vi "_Import Permanent Variable.vi"(7 "in":T3, 8 "error in (no error)":errorcluster, 9 "Array":path[](array[path]), 10 "section postfix":string, 11 "Path":path) -> (0 "error out":errorcluster, 5 "out":T3)   [LabVIEW 2017, in "INI-Static-Variable-Support.lvlib" / "CSM-Static-Variable-Manager.lvclass"]
uses:
  CSM-Static-Variable-Manager.lvclass
  LabVIEW-Config/Config.ctl
  LabVIEW-Config/LineToken.ctl
  LabVIEW-Config/LabVIEW-Config.lvlib
  <userlib>/_NEVSTOP/Communicable State Machine(CSM)/addons/API-String-Arugments-Support/API String Arguments Support.lvlib
  <userlib>/_NEVSTOP/Communicable State Machine(CSM)/_Shared/CSM Shared.lvlib
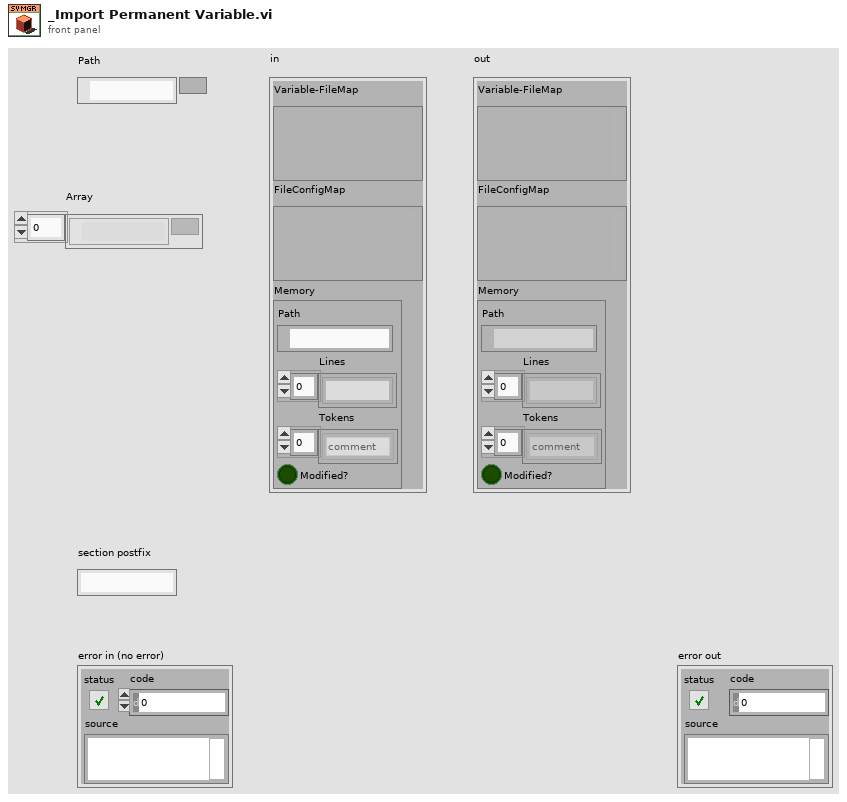
[diagram p1: front panel]
types:
  T1 = typedef "LabVIEW-Config.lvlib/Config.ctl" = cluster{"Path":path, "Lines":string[], "Tokens":T2[], "Modified?":bool}
  T2 = typedef "LabVIEW-Config.lvlib/LineToken.ctl" = enum8{"comment", "section", "key", "more"}
  T3 = cluster{"Variable-FileMap":variant, "FileConfigMap":variant, "Memory":T1}
  T4 = enum16{"Absolute path", "Relative path", "Not-a-path"}
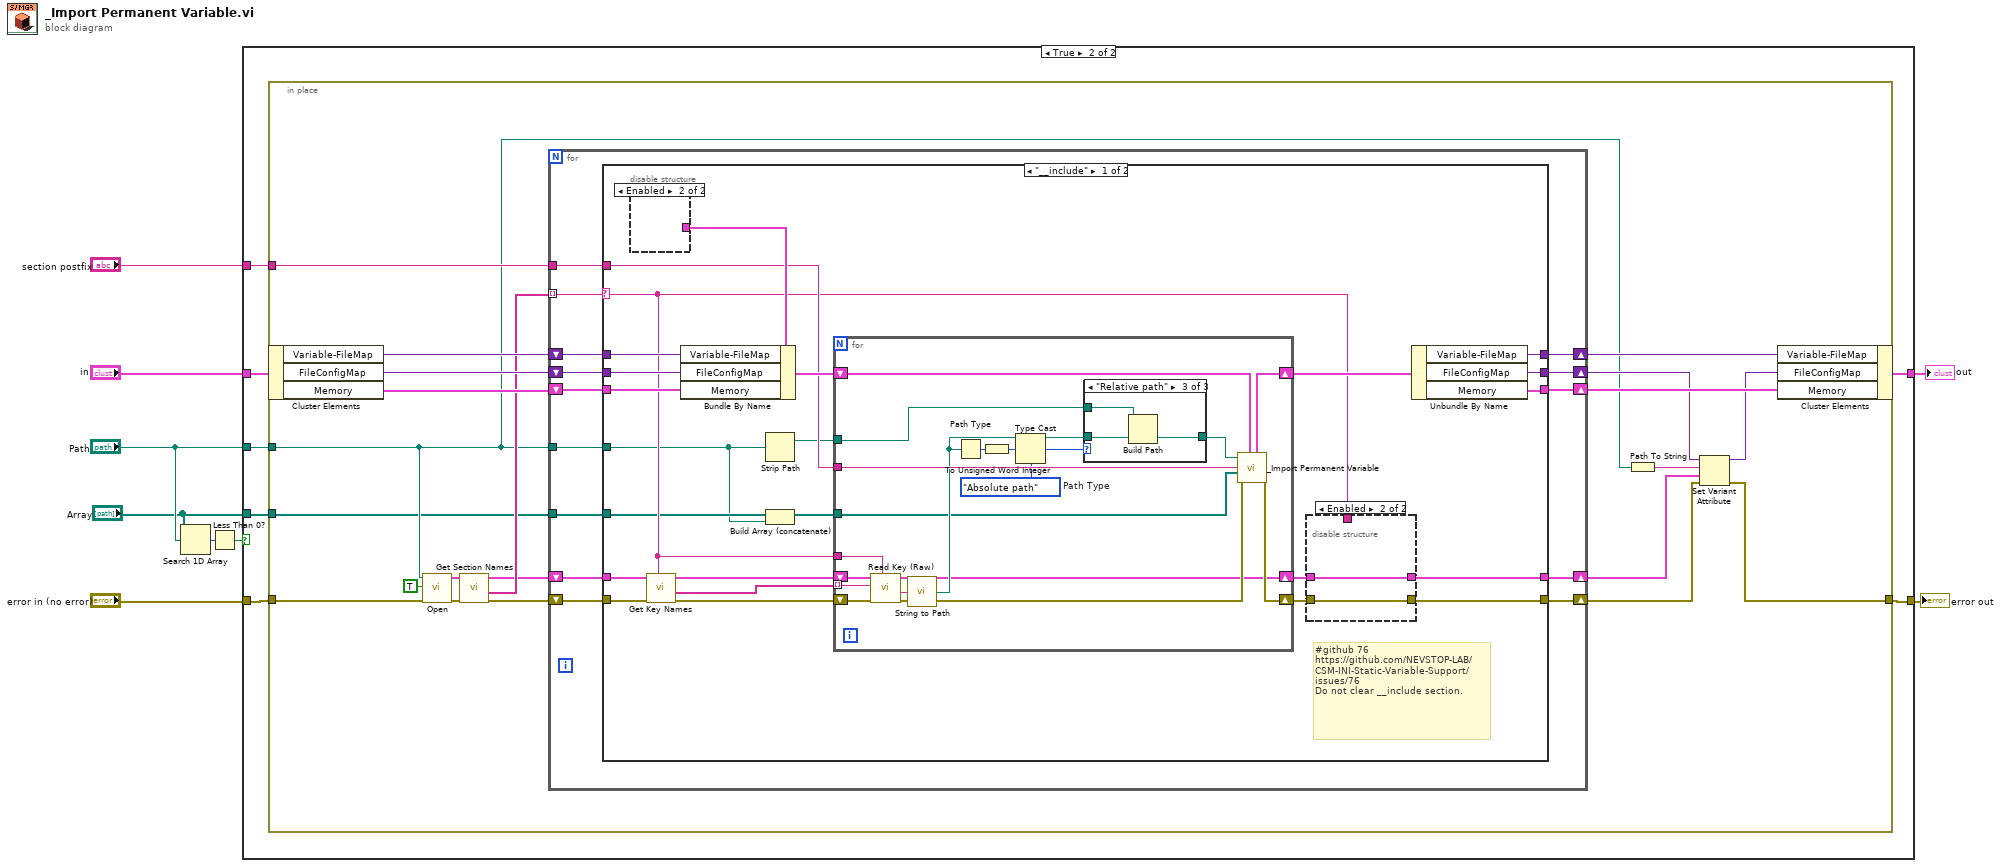
[diagram p0: block diagram]
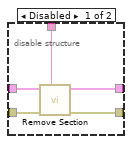
[diagram p3: hidden frame]
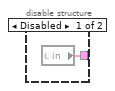
[diagram p6: hidden frame]
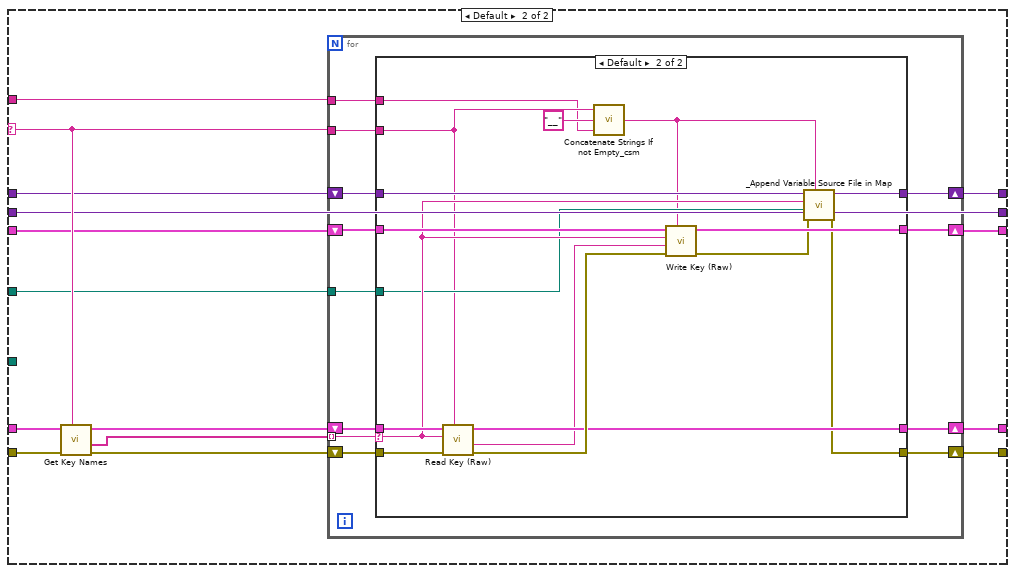
[diagram p7: hidden frame]
diagram:
  n1 = Search 1D Array(1D array="Array", element="Path") -> (index of element=w3:i32)  [unwired: 1 in]
  n2 = Less Than 0?(x=w3) -> (x < 0?=w2:bool)
  n3 = case shown="True" w2 {
    tunnel: "Path" -> [_ w18]
    tunnel: [w10 w17] -> w8
    tunnel: "section postfix" -> [_ w16]
    tunnel: "in" -> [w11 w15]
    tunnel: [w11 w14] -> w5
    tunnel: "error in (no error)" -> [w10 w13]
    tunnel: "Array" -> [_ w12]
    frame False {
    }
    frame True {
      n4 = in-place {
        in-place-border: w18 -> [w20]
        in-place-border: [w28] -> w17
        in-place-border: w16 -> [w39]
        in-place-border: w13 -> [w25]
        in-place-border: w12 -> [w19]
        n5 = in-place-cluster #1(w15) -> ("Variable-FileMap"=w38:variant, "FileConfigMap"=w34:variant, "Memory"=w37:T1)
        n6 = call "Open.vi"("error in (no error)"=w25, "Create if not exists? (T)"=TRUE, "Path"=w20) -> ("error out"=w27:errorcluster, "Config"=w26:T1)  [unwired: 5 in, 2 out]
        n7 = call "Get Section Names.vi"("error in (no error)"=w27, "Config in"=w26) -> ("error out"=w23:errorcluster, "Section Names"=w22:string[], "Config out"=w21:T1)  [unwired: 7 in]
        n8 = for {
          tunnel: w22 -> [w51] mode=indexing
          shift-right: [w49] -> w35
          shift-left: w37 -> [w50]
          shift-right: [w48] -> w29
          shift-left: w23 -> [w52]
          shift-right: [w47] -> w30
          shift-left: w21 -> [w53]
          shift-right: [w46] -> w36
          shift-left: w38 -> [w45]
          tunnel: w20 -> [w44]
          tunnel: w39 -> [w43]
          shift-right: [w42] -> w32
          shift-left: w34 -> [w41]
          tunnel: w19 -> [w40]
          n9 = case shown="\"__include\"" w51 {
            selector: w51 -> [w57 w122]
            tunnel: w53 -> [w65 w124]
            tunnel: w52 -> [w66 w123]
            tunnel: w50 -> [w73 w118]
            tunnel: [w70 w117] -> w49
            tunnel: [w60 w116] -> w48
            tunnel: [w58 w115] -> w47
            tunnel: [w68 w114] -> w46
            tunnel: w45 -> [w75 w113]
            tunnel: w44 -> [w54 w112]
            tunnel: w43 -> [w67 w111]
            tunnel: [w69 w110] -> w42
            tunnel: w41 -> [w74 w110]
            tunnel: w40 -> [w56 _]
            frame "__include" {
              # "#github 76\nhttps://github.com/NEVSTOP-LAB/CSM-INI-Static-Variable-Support/issues/76\nDo not clear __include section."
              n10 = disable-structure shown="Enabled" {
                disable-tunnel: [w109 _] -> w76
                frame Disabled {
                  n11 = local read "in"() -> (w109:T3)
                }
                frame Enabled {
                }
              }
              n12 = call "Get Key Names.vi"("Section Name"=w57, "error in (no error)"=w66, "Config in"=w65) -> ("error out"=w63:errorcluster, "Key Names"=w61:string[], "Config out"=w64:T1)  [unwired: 5 in, 1 out]
              n13 = Bundle By Name(cluster=w76, "Variable-FileMap"=w75, "FileConfigMap"=w74, "Memory"=w73) -> (w72:T3)
              n14 = Strip Path(path=w54) -> (stripped path=w62:path)  [unwired: 1 out]
              n15 = Build Array (concatenate)(w56, w54) -> (w55:path[])
              n16 = for {
                tunnel: w67 -> [w100]
                shift-right: [w103] -> w77
                shift-left: w63 -> [w96]
                shift-right: [w101] -> w71
                shift-left: w72 -> [w102]
                shift-right: [w91] -> w59
                shift-left: w64 -> [w97]
                tunnel: w62 -> [w98]
                tunnel: w61 -> [w95] mode=indexing
                tunnel: w57 -> [w90]
                tunnel: w55 -> [w89]
                w87 = T4."Absolute path"  # Path Type
                n17 = call "Read Key (Raw).vi"("Section Name"=w90, "error in (no error)"=w96, "Key Name"=w95, "Config in"=w97) -> ("error out"=w94:errorcluster, "Content"=w93:string, "Config out"=w91:T1)  [unwired: 4 in, 1 out]
                n18 = call <userlib>:"String to Path.vi"("String"=w93) -> ("Path"=w92:path)
                n19 = Path Type(1:w92) -> (0:w88:i16)
                n20 = To Unsigned Word Integer(number=w88) -> (unsigned 16bit integer=w86:u16)
                n21 = Type Cast(type=w87, x=w86) -> (*(type *) &x=w85:T4)
                n22 = case shown="\"Relative path\"" w85 {
                  tunnel: w92 -> [w104 w105 w107]
                  tunnel: [w104 w105 w106] -> w99
                  tunnel: w98 -> [_ _ w108]
                  frame "Absolute path" {
                  }
                  frame "Not-a-path" {
                  }
                  frame "Relative path" {
                    n23 = Build Path(base path=w108, name or relative path=w107) -> (appended path=w106:path)
                  }
                }
                n24 = call "_Import Permanent Variable.vi"("in"=w102, "error in (no error)"=w94, "Array"=w89, "section postfix"=w100, "Path"=w99) -> ("error out"=w103:errorcluster, "out"=w101:T3)  [unwired: 5 in]
              }
              n25 = disable-structure shown="Enabled" {
                disable-tunnel: w77 -> [w82 w83]
                disable-tunnel: [w81 w83] -> w60
                disable-tunnel: w59 -> [w80 w84]
                disable-tunnel: [w79 w84] -> w58
                disable-tunnel: w57 -> [w78 _]
                frame Disabled {
                  n26 = call "Remove Section.vi"("Section Name"=w78, "error in (no error)"=w82, "Config in"=w80) -> ("error out"=w81:errorcluster, "Config out"=w79:T1)  [unwired: 6 in, 1 out]
                }
                frame Enabled {
                }
              }
              n27 = Unbundle By Name(w71) -> ("Variable-FileMap"=w68:variant, "FileConfigMap"=w69:variant, "Memory"=w70:T1)
            }
            frame Default {
              n28 = call "Get Key Names.vi"("Section Name"=w122, "error in (no error)"=w123, "Config in"=w124) -> ("error out"=w119:errorcluster, "Key Names"=w120:string[], "Config out"=w121:T1)  [unwired: 5 in, 1 out]
              n29 = for {
                tunnel: w122 -> [w126]
                tunnel: w120 -> [w128] mode=indexing
                shift-right: [w130] -> w116
                shift-left: w119 -> [w135]
                shift-right: [w134] -> w117
                shift-left: w118 -> [w133]
                shift-right: [w132] -> w115
                shift-left: w121 -> [w136]
                shift-right: [w131] -> w114
                shift-left: w113 -> [w129]
                tunnel: w112 -> [w127]
                tunnel: w111 -> [w125]
                n30 = case shown="Default" w128 {
                  selector: w128 -> [_ w146]
                  tunnel: w136 -> [w138 w157]
                  tunnel: w135 -> [w137 w156]
                  tunnel: [w139 w155] -> w134
                  tunnel: w133 -> [w139 w154]
                  tunnel: [w138 w152] -> w132
                  tunnel: [w140 w151] -> w131
                  tunnel: [w137 w149] -> w130
                  tunnel: w129 -> [w140 w148]
                  tunnel: w127 -> [_ w145]
                  tunnel: w126 -> [_ w142]
                  tunnel: w125 -> [_ w141]
                  frame "Core.Current VI Reference" {
                  }
                  frame Default {
                    n31 = call "Read Key (Raw).vi"("Section Name"=w142, "error in (no error)"=w156, "Key Name"=w146, "Config in"=w157) -> ("error out"=w153:errorcluster, "Content"=w147:string, "Config out"=w152:T1)  [unwired: 4 in, 1 out]
                    n32 = call <userlib>:"Concatenate Strings If not Empty_csm.vi"("String"=w141, "seperator(:)"="__", "prefix"=w142) -> ("result"=w144:string)  [unwired: 2 in]
                    n33 = call "Write Key (Raw).vi"("Section Name"=w144, "error in (no error)"=w153, "Content"=w147, "Key Name"=w146, "Config in"=w154) -> ("error out"=w150:errorcluster, "Config out"=w155:T1)  [unwired: 4 in, 1 out]
                    n34 = call "_Append Variable Source File in Map.vi"("String"=w144, "error in (no error)"=w150, "dup path"=w145, "Content"=w146, "Variable-FileMap"=w148) -> ("error out"=w149:errorcluster, "Variant"=w151:variant)  [unwired: 5 in]
                  }
                }
              }
            }
          }
        }
        n35 = Path To String(path=w20) -> (string=w33:string)
        n36 = Set Variant Attribute(Variant=w32, name=w33, value=w30, error in=w29) -> (Variant out=w31:variant, error out=w28:errorcluster)  [unwired: 1 out]
        n37 = in-place-cluster #1("Variable-FileMap"=w36, "FileConfigMap"=w31, "Memory"=w35) -> (w14:T3)
      }
    }
  }
  "error out" <- w8
  "out" <- w5
